vi "h_generation.vi"(1 "every_mean_points":dbl[](array[numeric]), 2 "Y":dbl[](array[numeric])) -> (0 "h(t)":dbl[](array[numeric]))   [LabVIEW 2018]
panel:
  out "h1(t)":dbl[](array[numeric])
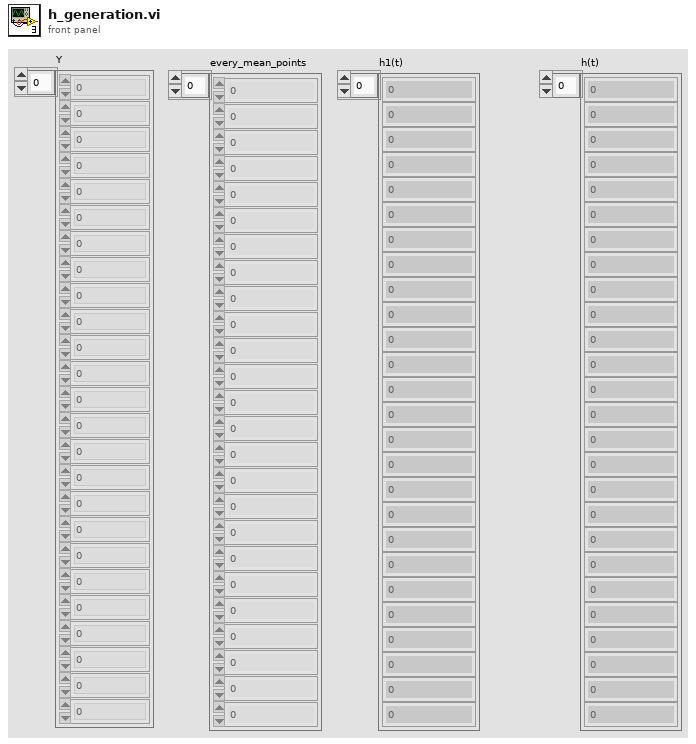
[diagram p1: front panel]
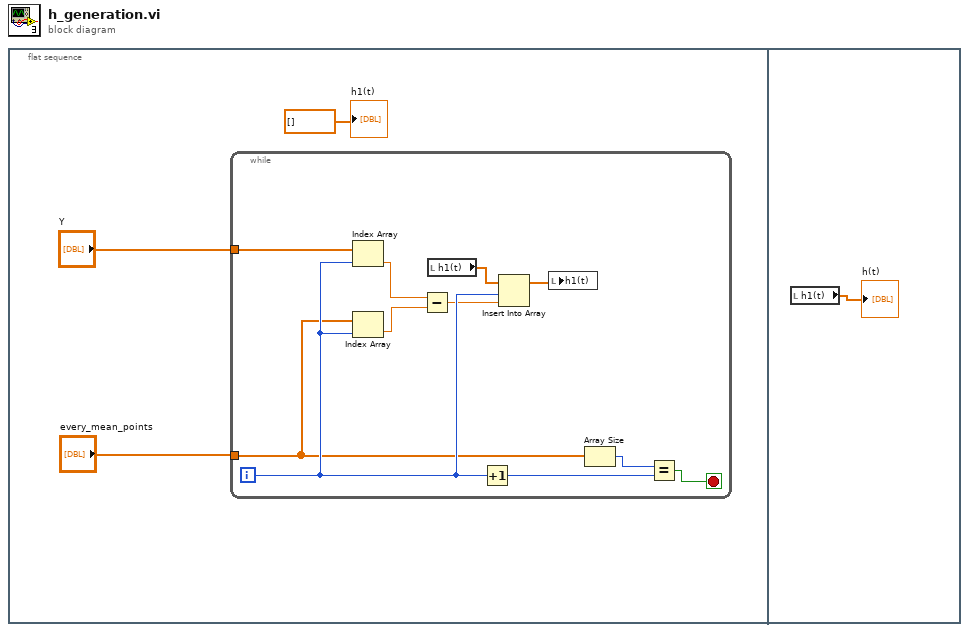
[diagram p0: block diagram]
diagram:
  n1 = flat-sequence {
    frame #0 {
      n2 = while {
        tunnel: "Y" -> [w11]
        tunnel: "every_mean_points" -> [w5]
        i -> [w9]
        stop <- w12 stop-if-true
        n3 = Index Array(array=w11, index=w9) -> (element=w10:dbl)
        n4 = Index Array(array=w5, index=w9) -> (element=w4:dbl)
        n5 = Subtract(x=w10, y=w4) -> (x-y=w8:dbl)
        n6 = local read "h1(t)"() -> (w6:dbl[])
        n7 = Increment(x=w9) -> (x+1=w13:i32)
        n8 = Insert Into Array(array=w6, index=w9, new element=w8) -> (w7:dbl[])
        n9 = local write "h1(t)"(w7) -> ()
        n10 = Array Size(array=w5) -> (size(s)=w14:i32)
        n11 = Equal?(x=w14, y=w13) -> (x = y?=w12:bool)
      }
      "h1(t)" <- dbl[] []
    }
    frame #1 {
      n12 = local read "h1(t)"() -> (→"h(t)":dbl[])
    }
  }
